vi "MSEncoder Case-3-LaserTrig.vi"(8 "error in (no error)":errorcluster, 9 "ParamValIn":variant, 11 "MSEncoder in":refnum<class "MSEncoder.lvclass">) -> (0 "error out":errorcluster, 3 "MSEncoder out":refnum<class "MSEncoder.lvclass">)   [LabVIEW 2018, in "MSEncoder.lvclass"]
uses:
  MSEncoder.lvclass
  Ctl/MSEditorParam laserTrig.ctl
  MSEncoder.lvclass/MSEncoder.ctl
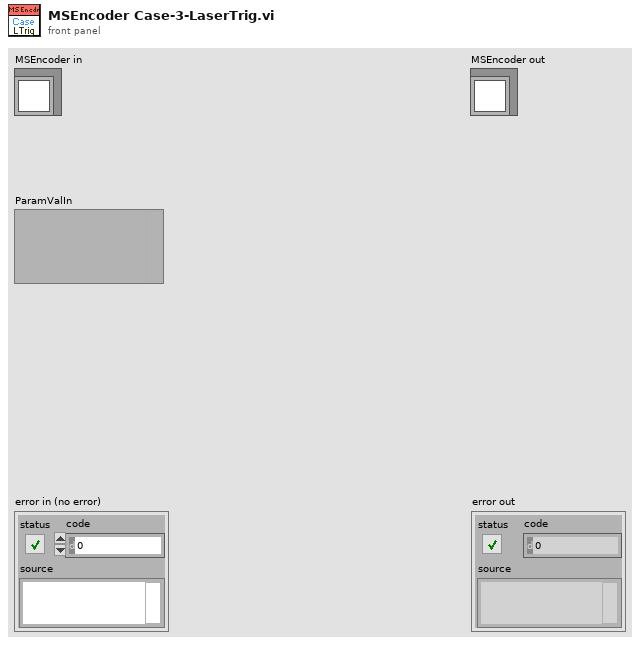
[diagram p1: front panel]
types:
  T1 = typedef "MSEditorParam laserTrig.ctl" = cluster{"trigFreq":ext, "phaseDeg":ext, "shots":u32}
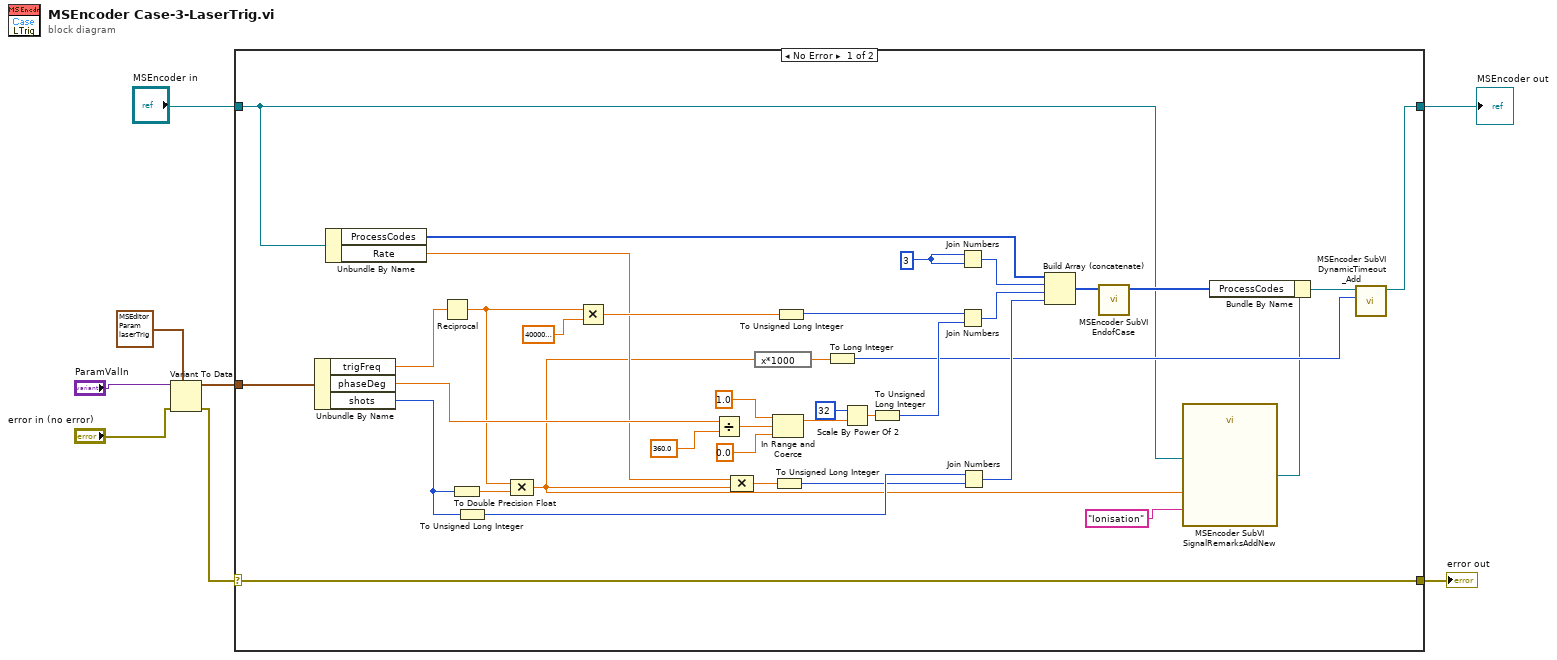
[diagram p0: block diagram]
diagram:
  n1 = Variant To Data(error in="error in (no error)", type=T1 {"trigFreq"=100.0, "phaseDeg"=90.0, "shots"=1} ("ParamValueType"), Variant="ParamValIn") -> (data=w2:T1, error out=w1:errorcluster)
  n2 = case shown="No Error" w1 {
    selector: w1 -> [w44 w47]
    tunnel: "MSEncoder in" -> [w13 w46]
    tunnel: [w44 w47] -> w8
    tunnel: [w16 w46] -> w6
    tunnel: w2 -> [w21 _]
    frame No Error {
      w33 = u32 3
      n3 = Unbundle By Name(w21) -> ("trigFreq"=w42:ext, "phaseDeg"=w41:ext, "shots"=w40:u32)
      n4 = Unbundle By Name(w13) -> ("ProcessCodes"=w14:u64[], "Rate"=w20:dbl)
      n5 = Reciprocal(x=w42) -> (1/x=w23:ext)
      n6 = To Double Precision Float(number=w40) -> (double precision float=w18:dbl)
      n7 = To Unsigned Long Integer(number=w40) -> (unsigned 32bit integer=w25:u32)
      n8 = Compound Arithmetic op=MULTIPLY(w23, w18) -> (w10:ext)
      n9 = Multiply(x=w23, y=40000000.0) -> (x*y=w29:ext)
      n10 = Divide(x=w41, y=360.0) -> (x/y=w39:ext)
      n11 = Compound Arithmetic op=MULTIPLY(w20, w10) -> (w19:ext)
      n12 = expression code="x*1000"(w10) -> (w17:ext)
      n13 = In Range and Coerce(upper limit=1.0, x=w39, lower limit=0.0) -> (coerced(x)=w36:ext)  [unwired: 1 out]
      n14 = To Unsigned Long Integer(number=w19) -> (unsigned 32bit integer=w22:u32)
      n15 = To Unsigned Long Integer(number=w29) -> (unsigned 32bit integer=w26:u32)
      n16 = To Long Integer(number=w17) -> (32bit integer=w15:i32)
      n17 = Scale By Power Of 2(n=i16 32, x=w36) -> (x*2^n=w34:ext)
      n18 = To Unsigned Long Integer(number=w34) -> (unsigned 32bit integer=w28:u32)
      n19 = Join Numbers(hi=w33, lo=w33) -> ((hi.lo)=w32:u64)
      n20 = Join Numbers(hi=w26, lo=w28) -> ((hi.lo)=w27:u64)
      n21 = Join Numbers(hi=w25, lo=w22) -> ((hi.lo)=w24:u64)
      n22 = Build Array (concatenate)(w14, w32, w27, w24) -> (w45:u64[])
      n23 = call "MSEncoder SubVI EndofCase.vi"("Case codes"=w45) -> ("Case codes with end"=w43:u64[])  [unwired: 9 in, 1 out]
      n24 = call "MSEncoder SubVI SignalRemarksAddNew.vi"("Label"="Ionisation", "Scan time"=w10, "MSEncoder in"=w13) -> ("MSEncoder out"=w12:refnum<class "MSEncoder.lvclass">)  [unwired: 7 in, 1 out]
      n25 = Bundle By Name(cluster=w12, "ProcessCodes"=w43) -> (w11:refnum<class "MSEncoder.lvclass">)
      n26 = call "MSEncoder SubVI DynamicTimeout_Add.vi"("Timeout_ms"=w15, "MSEncoder"=w11) -> ("MSEncoder"=w16:refnum<class "MSEncoder.lvclass">)  [unwired: 8 in, 1 out]
    }
    frame Error {
    }
  }
  "error out" <- w8
  "MSEncoder out" <- w6
